vi "set number of steps to move.vi"(8 "error in":errorcluster, 9 "axis (def: fine)":enum16{"fine", "coarse"}(ring), 10 "number of steps to set":dbl, 11 "GPIB # (in): def. 6":string="6") -> (0 "error out":errorcluster, 3 "GPIB # (out)":string)   [LabVIEW 2009]
uses:
  mc2mc4.llb/MC2/4  SendCommand.VI
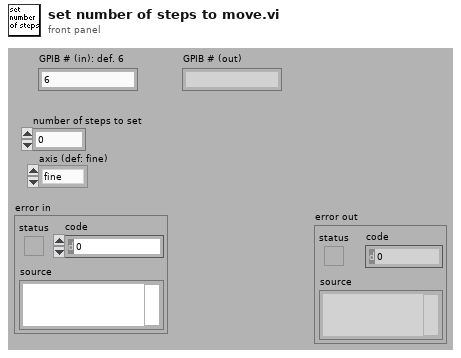
[diagram p1: front panel]
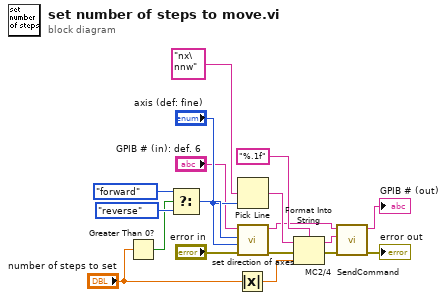
[diagram p0: block diagram]
diagram:
  n1 = Greater Than 0?(x="number of steps to set") -> (x > 0?=w13:bool)
  n2 = Select(t=enum16{"forward", "reverse"}."forward" ("direction (def: forward)"), s=w13, f=enum16{"forward", "reverse"}."reverse" ("direction (def: forward)")) -> (s? t:f=w12:enum16{"forward", "reverse"})
  n3 = Absolute Value(x="number of steps to set") -> (abs(x)=w10:dbl)
  n4 = Pick Line(multi-line string="nx\nnw", line index="axis (def: fine)") -> (output string=w6:string)  [unwired: 1 out]
  n5 = call "set direction of axes.vi"("error in"="error in", "stage to move (def: fine)"="axis (def: fine)", "direction (def: forward)"=w12, "GPIB # (in): def. 6"="GPIB # (in): def. 6") -> ("error out"=w8:errorcluster, "GPIB # (out)"=w2:string)  [unwired: 6 out]
  n6 = Format Into String ("Set number of\n Big Steps")(format string="%.1f", initial string=w6, error in=w8, w10) -> (resulting string=w17:string, error out=w16:errorcluster)
  n7 = call "MC2/4  SendCommand.VI"("error in (no error)"=w16, "MC2 / MC4 Command"=w17, "GPIB # (in): def.6"=w2) -> ("error out"=→"error out":errorcluster, "GPIB # (out)"=→"GPIB # (out)":string)  [unwired: 7 out]
